vi "Write Configuration.vi"(8 "error in (no error)":errorcluster, 11 "Report Generator In":refnum<class "Report Generator.lvclass">) -> (0 "error out":errorcluster, 3 "Report Generator Out":refnum<class "Report Generator.lvclass">)   [LabVIEW 2020, in "Report Generator.lvclass"]
doc: "Method that write the object attributes to config file."
uses:
  Report Generator.lvclass
  C:/Users/anton/Documents/GitHub/LUnit/source/Application Framework/Process Classes/Process/Process.lvclass
  Report Generator.lvclass/Report Generator.ctl
  Application Framework/Process Classes/Process/Process.lvclass
  Report Classes/Test Report/Test Report.lvclass
  Application Framework/Support/Configuration File/Configuration File.lvlib
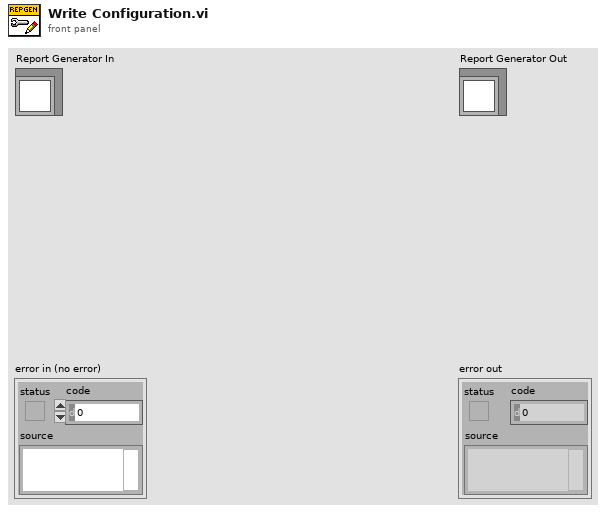
[diagram p1: front panel]
types:
  T1 = typedef "NI_LVConfig.lvlib/Config Data RefNum.ctl" = refnum<k1>
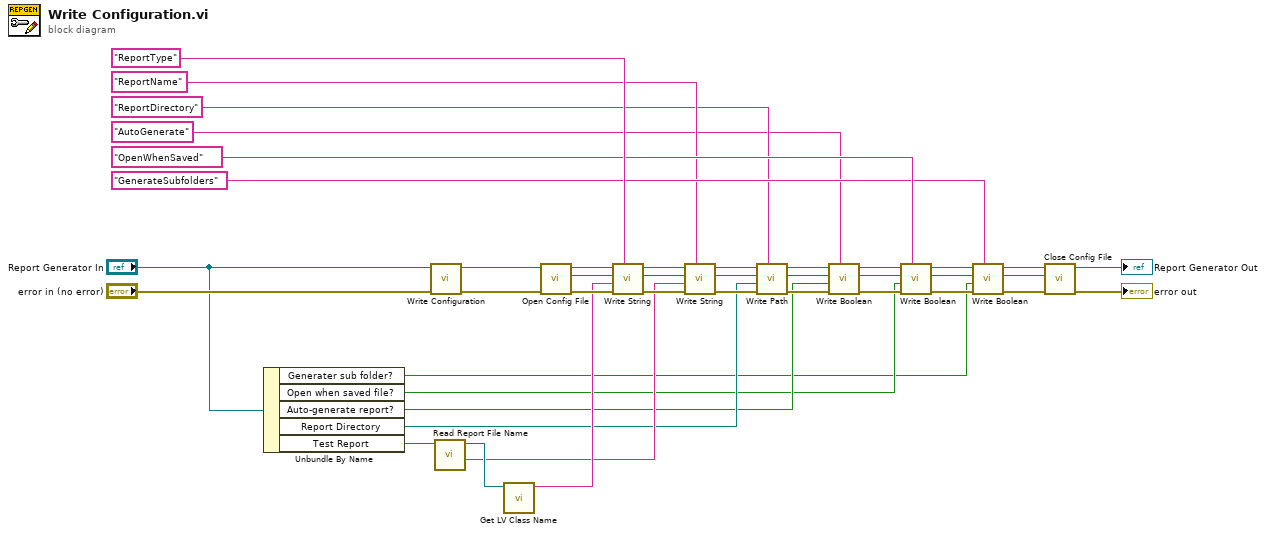
[diagram p0: block diagram]
diagram:
  n1 = Unbundle By Name("Report Generator In") -> ("Generater sub folder?"=w1:bool, "Open when saved file?"=w2:bool, "Auto-generate report?"=w3:bool, "Report Directory"=w7:path, "Test Report"=w11:refnum<class "Test Report.lvclass">)
  n2 = call-parent "Write Configuration.vi"("error in (no error)"="error in (no error)", "Process In"="Report Generator In") -> ("error out"=w18:errorcluster, "Process Out"=w19:refnum<class "Report Generator.lvclass">)  [unwired: 8 in]
  n3 = call-dynamic "Read Report File Name.vi"("Report In"=w11) -> ("Report File Name without extension"=w8:string, "Report Out"=w9:refnum<class "Test Report.lvclass">)  [unwired: 7 in, 2 out]
  n4 = call <vilib>:"Get LV Class Name.vi"("object"=w9) -> ("class name"=w10:string)  [unwired: 9 in, 1 out]
  n5 = call "Open Config File.vi"("error in (no error)"=w18, "Process in"=w19) -> ("error out"=w36:errorcluster, "refnum out"=w25:T1, "Process out"=w37:refnum<class "Report Generator.lvclass">)  [unwired: 6 in, 1 out]
  n6 = call "Write String.vi"("key"="ReportType", "error in (no error)"=w36, "default value"=w10, "refnum"=w25, "Process in"=w37) -> ("error out"=w34:errorcluster, "refnum out"=w24:T1, "Process out"=w35:refnum<class "Report Generator.lvclass">)  [unwired: 4 in]
  n7 = call "Write String.vi"("key"="ReportName", "error in (no error)"=w34, "default value"=w8, "refnum"=w24, "Process in"=w35) -> ("error out"=w32:errorcluster, "refnum out"=w23:T1, "Process out"=w33:refnum<class "Report Generator.lvclass">)  [unwired: 4 in]
  n8 = call "Write Path.vi"("key"="ReportDirectory", "error in (no error)"=w32, "default value"=w7, "refnum"=w23, "Process in"=w33) -> ("error out"=w30:errorcluster, "refnum out"=w22:T1, "Process out"=w31:refnum<class "Report Generator.lvclass">)  [unwired: 4 in]
  n9 = call "Write Boolean.vi"("key"="AutoGenerate", "error in (no error)"=w30, "default value"=w3, "refnum"=w22, "Process in"=w31) -> ("error out"=w28:errorcluster, "refnum out"=w21:T1, "Process out"=w29:refnum<class "Report Generator.lvclass">)  [unwired: 4 in]
  n10 = call "Write Boolean.vi"("key"="OpenWhenSaved", "error in (no error)"=w28, "default value"=w2, "refnum"=w21, "Process in"=w29) -> ("error out"=w26:errorcluster, "refnum out"=w20:T1, "Process out"=w27:refnum<class "Report Generator.lvclass">)  [unwired: 4 in]
  n11 = call "Write Boolean.vi"("key"="GenerateSubfolders", "error in (no error)"=w26, "default value"=w1, "refnum"=w20, "Process in"=w27) -> ("error out"=w40:errorcluster, "refnum out"=w39:T1, "Process out"=w38:refnum<class "Report Generator.lvclass">)  [unwired: 4 in]
  n12 = call "Close Config File.vi"("error in (no error)"=w40, "refnum"=w39, "Process in"=w38) -> ("error out"=→"error out":errorcluster, "Process out"=→"Report Generator Out":refnum<class "Report Generator.lvclass">)  [unwired: 6 in, 1 out]
